vi "task.mode_lua.vi"(5 "LuaVIEW reference":T1) -> (15 "error out":errorcluster)   [LabVIEW 2012]
doc: "Returns the mode of the specified task or, when no argument is passed, the mode of the calling task.\nParameters:\n[str:task_identifier]\nResults:\nstr:mode\nErrors:\nNo such task."
uses:
  typedefs/t_LuaVIEW Reference.ctl
  typedefs/t_LuaVIEW Task List Methods.ctl
  typedefs/t_LuaVIEW Task State Methods.ctl
  subvis/private/LuaVIEW Push (string).vi
  subvis/private/LuaVIEW Pull (string).vi
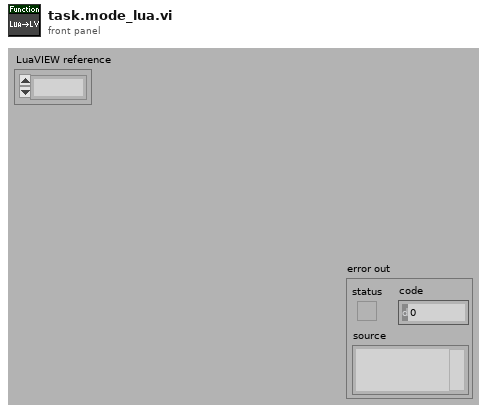
[diagram p1: front panel]
types:
  T1 = typedef "t_LuaVIEW Reference.ctl" = refnum<k1>
  T2 = typedef "t_LuaVIEW Task List Methods.ctl" = enum16{"clear list", "add", "test", "remove", "get ref", "get task info", "get list", "get script info", "ongoing?", "resume", "pause", "stop", "confirm", "message"}
  T3 = typedef "t_LuaVIEW Task State Methods.ctl" = enum16{"cleanup", "set initial", "set mode", "set active mode", "set error", "get task info", "get script info", "set signal", "clear signal", "test handled", "test delegated", "test signal", "handle signal", "delegate signal", "allow signal", "disallow signal", "disallow all", "signals?", "delegated signals?", "protection++", "protection--", "protection=0", "message", "next message", "pop message", "message available?", "force stop", "set swap preps", "apply swap preps"}
  T4 = typedef "LuaVIEW Task Info.ctl" = cluster{"main script":string, "identifier":string, "class":string, "description":string, "mode":T5, "handler":string, "LuaVIEW reference":T1, "scripts":i32, "hide":bool, "active":bool, "error msg":string, "defer":bool, "launch":enum16{"asynchronous", "manual", "synchronous"}, "main path valid":bool, "start time":dbl, "swap time":dbl, "task VI":refnum<vi>, "prefsys":enum32{"invalid execution system", "user interface", "standard", "instrument i/o", "data acquisition", "other 1", "other 2", "same as caller"}, "priority":enum32{"invalid priority", "background priority", "normal priority", "above normal priority", "high priority", "time critical priority", "subroutine"}, "signal flags":u32, "allow mask":u32, "handle mask":u32, "disallow manual":bool}
  T5 = typedef "t_LuaVIEW Task Modes.ctl" = enum16{"initializing", "running", "executing", "paused", "error", "swapping"}
  T6 = typedef "t_LuaVIEW Task State Pane.ctl" = refnum<vi>
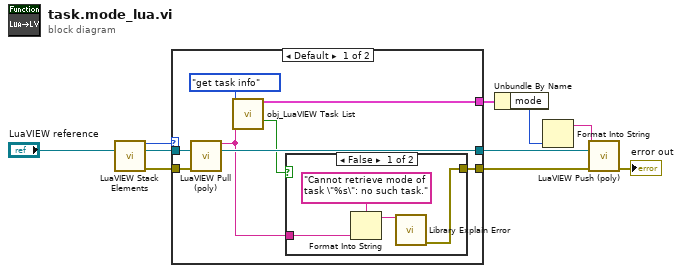
[diagram p0: block diagram]
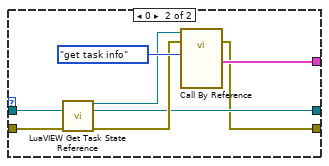
[diagram p3: hidden frame]
diagram:
  n1 = call "LuaVIEW Stack Elements.vi"("LuaVIEW reference in"="LuaVIEW reference") -> ("elements"=w4:i32, "LuaVIEW reference out"=w6:T1, "error out"=w5:errorcluster)  [unwired: 12 in]
  n2 = case shown="Default" w4 {
    tunnel: w6 -> [w17 w30]
    tunnel: w5 -> [w18 w29]
    tunnel: [w14 w25] -> w3
    tunnel: [w15 w24] -> w2
    tunnel: [w12 w23] -> w1
    frame Default {
      n3 = call-poly "LuaVIEW Pull (poly).vi"("LuaVIEW reference in"=w17, "error in (no error)"=w18) -> ("string"=w11:string, "LuaVIEW reference out"=w15:T1)  [unwired: 11 in, 1 out]
      n4 = call "obj_LuaVIEW Task List.vi"("method"=t_LuaVIEW_Task_List_Methods."get task info", "task identifier"=w11) -> ("task info"=w14:T4, "set/ongoing"=w13:bool)  [unwired: 8 in, 4 out]
      n5 = case shown="False" w13 {
        tunnel: [w22 _] -> w12
        tunnel: w11 -> [w21 _]
        frame False {
          n6 = Format Into String(format string="Cannot retrieve mode of task \"%s\": no such task.", w21) -> (resulting string=w19:string)  [unwired: 2 in, 1 out]
          n7 = call "Library Explain Error.vi"("explanation prefix (none)"=w19) -> ("explained error"=w22:errorcluster)  [unwired: 14 in]
        }
        frame True {
        }
      }
    }
    frame 0 {
      n8 = call "LuaVIEW Get Task State Reference.vi"("LuaVIEW reference in"=w30, "error in (no error)"=w29) -> ("task state reference"=w27:T6, "LuaVIEW reference out"=w24:T1, "error out"=w26:errorcluster)  [unwired: 11 in]
      n9 = call-by-ref "?"(reference=w27, error in=w26, "method"=t_LuaVIEW_Task_State_Methods."get task info") -> (error out=w23:errorcluster, "task info {get task info}"=w25:T4)  [unwired: 10 in, 5 out]
    }
  }
  n10 = Unbundle By Name(w3) -> ("mode"=w9:T5)
  n11 = Format Into String(w9) -> (resulting string=w8:string)  [unwired: 3 in, 1 out]
  n12 = call-poly "LuaVIEW Push (poly).vi"("string"=w8, "LuaVIEW reference in"=w2, "error in (no error)"=w1) -> ("error out"=→"error out":errorcluster)  [unwired: 11 in, 1 out]
